vi "UI_Defer Front Panel Updates.vi"(0 "This VI":refnum<vi>, 7 "Defer Panel Updates":bool=TRUE, 11 "error in (no error)":errorcluster) -> (15 "error out":errorcluster)   [LabVIEW 2021, in "CANOpen Addon System Explorer.lvlib"]
uses:
  CANOpen Addon System Explorer.lvlib
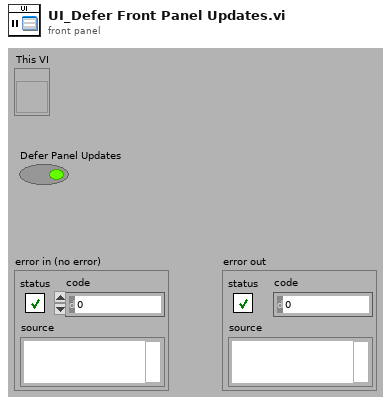
[diagram p1: front panel]
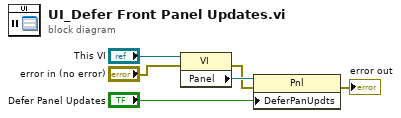
[diagram p0: block diagram]
diagram:
  n1 = property class="VI"(reference="This VI", error in="error in (no error)") -> (error out=w3:errorcluster, "Panel"=w5:refnum<vi>)  [unwired: 1 out]
  n2 = property class="Pnl"(reference=w5, error in=w3, "DeferPanUpdts"="Defer Panel Updates") -> (error out=→"error out":errorcluster)  [unwired: 1 out]
